vi "set odometer.vi"(10 "Odometer":i32(slide) scale=0.0..250.0, 11 "Array":T1[](array[typedef]) {"Data" format="%.0x"}) -> (3 "Array 2":T1[](array[typedef]) {"Data" format="%.0x"})   [LabVIEW 2021, in "uCanDriver.lvlib" / "uCAN.lvclass"]
uses:
  uCAN.lvclass
  typedefs/frame.ctl
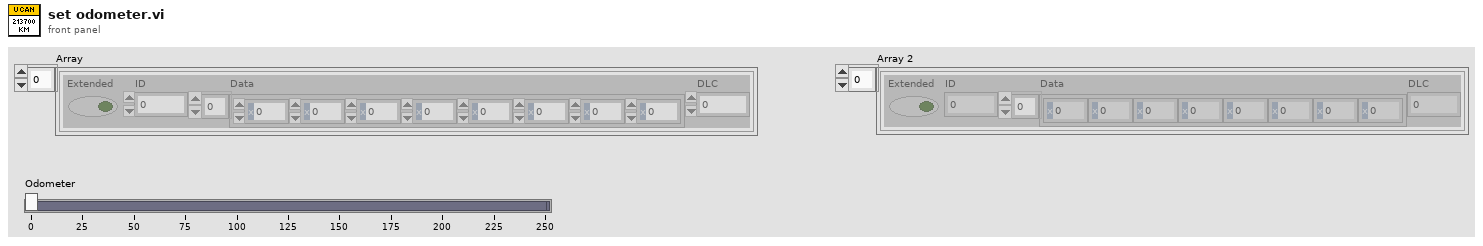
[diagram p1: front panel]
types:
  T1 = typedef "uCanDriver.lvlib/uCAN.lvclass/frame.ctl" = cluster{"Extended":bool, "ID":u32, "Data":u8[], "DLC":u8}
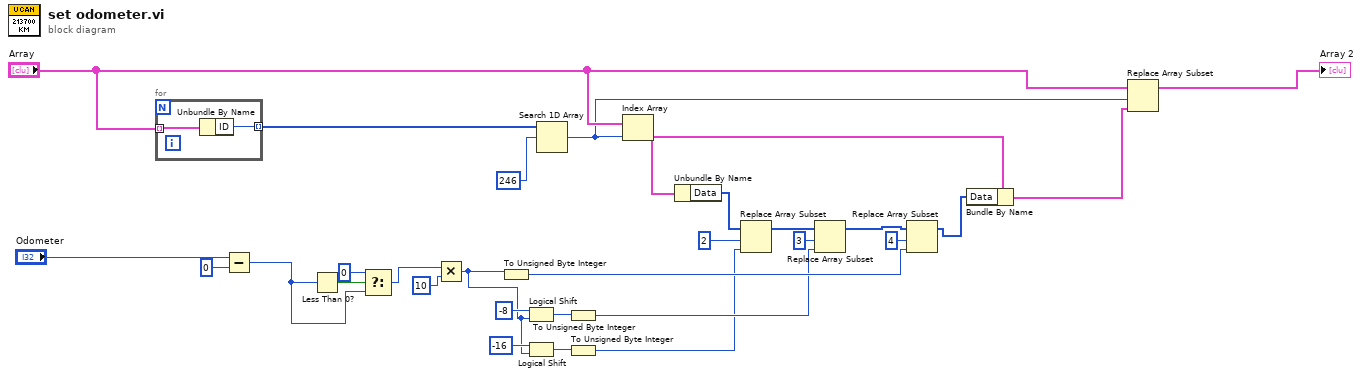
[diagram p0: block diagram]
diagram:
  n1 = for {
    tunnel: "Array" -> [w31] mode=indexing
    tunnel: [w30] -> w27 mode=indexing
    n2 = Unbundle By Name(w31) -> ("ID"=w30:u32)
  }
  n3 = Subtract(x="Odometer", y=u16 0) -> (x-y=w11:i32)
  n4 = Less Than 0?(x=w11) -> (x < 0?=w13:bool)
  n5 = Select(t=u16 0, s=w13, f=w11) -> (s? t:f=w10:i32)
  n6 = Multiply(x=w10, y=i16 10) -> (x*y=w1:i32)
  n7 = To Unsigned Byte Integer(number=w1) -> (unsigned 8bit integer=w4:u8)
  n8 = Logical Shift(y=i16 -8, x=w1) -> (x << y=w17:i32)
  n9 = Logical Shift(y=i16 -16, x=w1) -> (x << y=w6:i32)
  n10 = Search 1D Array(1D array=w27, element=u32 246) -> (index of element=w25:i32)  [unwired: 1 in]
  n11 = To Unsigned Byte Integer(number=w17) -> (unsigned 8bit integer=w3:u8)
  n12 = To Unsigned Byte Integer(number=w6) -> (unsigned 8bit integer=w2:u8)
  n13 = Index Array(array="Array", index=w25) -> (element=w29:T1)
  n14 = Unbundle By Name(w29) -> ("Data"=w21:u8[])
  n15 = Replace Array Subset(array=w21, new element=w2, index=2) -> (w20:u8[])
  n16 = Replace Array Subset(array=w20, new element=w3, index=3) -> (w7:u8[])
  n17 = Replace Array Subset(array=w7, new element=w4, index=4) -> (w8:u8[])
  n18 = Bundle By Name(cluster=w29, "Data"=w8) -> (w23:T1)
  n19 = Replace Array Subset(array="Array", new element=w23, index=w25) -> (→"Array 2":T1[])
